vi "native norm.vi"(10 "Vector":cluster{"X":sgl, "Y":sgl, "Z":sgl}) -> (2 "Norm":sgl)   [LabVIEW 2020]
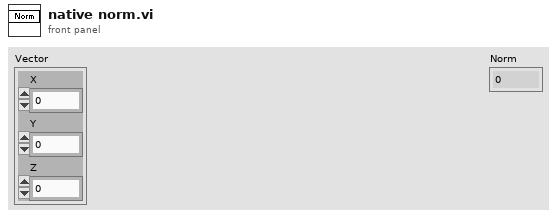
[diagram p1: front panel]
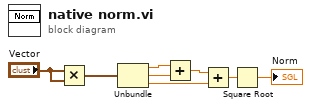
[diagram p0: block diagram]
diagram:
  n1 = Multiply(x="Vector", y="Vector") -> (x*y=w8:cluster{"X":sgl, "Y":sgl, "Z":sgl})
  n2 = Unbundle(w8) -> ("X"=w6:sgl, "Y"=w5:sgl, "Z"=w4:sgl)
  n3 = Add(x=w6, y=w5) -> (x+y=w3:sgl)
  n4 = Add(x=w3, y=w4) -> (x+y=w2:sgl)
  n5 = Square Root(x=w2) -> (sqrt(x)=→"Norm":sgl)
